vi "get_status_code_and_header_string.vi"(8 "error in (no error)":errorcluster, 11 "Request in":refnum<class "Request.lvclass">) -> (0 "error out":errorcluster, 1 "status_code":u16, 2 "headers":string, 3 "Request out":refnum<class "Request.lvclass">)   [LabVIEW 2020, in "HTTP Client reqwest.lvclass"]
uses:
  HTTP Client reqwest.lvclass
  HTTP Client reqwest.lvclass/HTTP Client reqwest.ctl
  Request/Request.lvclass
  Headers/Headers.lvclass
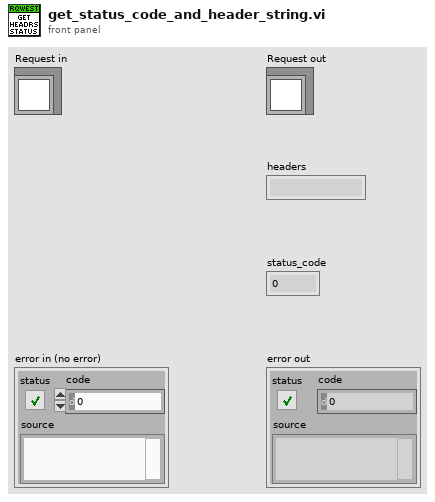
[diagram p1: front panel]
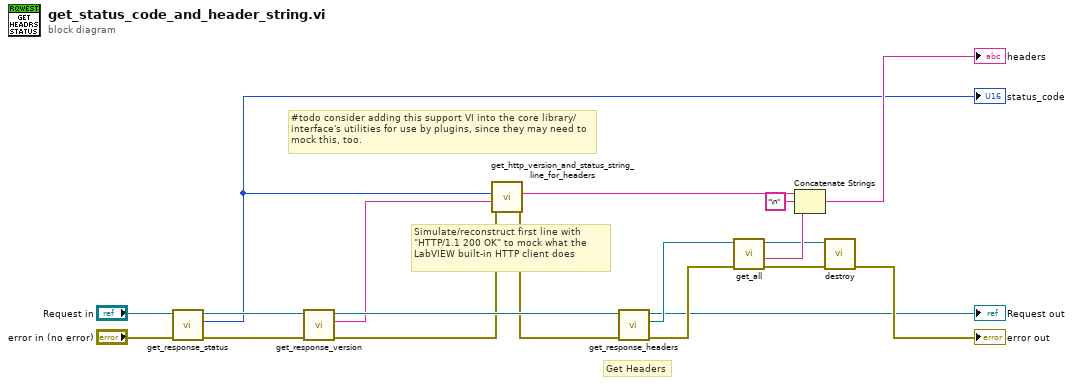
[diagram p0: block diagram]
diagram:
  # "#todo consider adding this support VI into the core library/interface's utilities for use by plugins, since they may need to mock this, too."
  # "Simulate/reconstruct first line with \"HTTP/1.1 200 OK\" to mock what the LabVIEW built-in HTTP client does"
  # "Get Headers"
  n1 = call "get_response_status.vi"("error in (no error)"="error in (no error)", "Request in"="Request in") -> ("error out"=w19:errorcluster, "status_code"=w2:u16, "Request out"=w18:refnum<class "Request.lvclass">)  [unwired: 7 in]
  "status_code" <- w2
  n2 = call "get_response_version.vi"("error in (no error)"=w19, "Request in"=w18) -> ("error out"=w5:errorcluster, "response_version"=w3:string, "Request in"=w12:refnum<class "Request.lvclass">)  [unwired: 7 in]
  n3 = call "get_http_version_and_status_string_line_for_headers.vi"("error in (no error)"=w5, "response_version"=w3, "status_code"=w2) -> ("error out"=w4:errorcluster, "http version and status string"=w1:string)  [unwired: 7 in]
  n4 = call "get_response_headers.vi"("error in (no error)"=w4, "Request in"=w12) -> ("error out"=w8:errorcluster, "response_headers"=w7:refnum<class "Headers.lvclass">, "Request in"=→"Request out":refnum<class "Request.lvclass">)  [unwired: 7 in]
  n5 = call "get_all.vi"("error in (no error)"=w8, "Headers in"=w7) -> ("error out"=w10:errorcluster, "headers"=w13:string, "Headers in"=w9:refnum<class "Headers.lvclass">)  [unwired: 6 in, 1 out]
  n6 = Concatenate Strings(w1, "\n" ("string"), w13) -> (→"headers":string)
  n7 = call "destroy.vi"("error in (no error)"=w10, "Headers in"=w9) -> ("error out"=→"error out":errorcluster)  [unwired: 9 in]
